vi "parse url.vi"(11 "connection string in":string) -> (1 "service":string, 2 "port":u16, 3 "net address":u32)   [LabVIEW 2015]
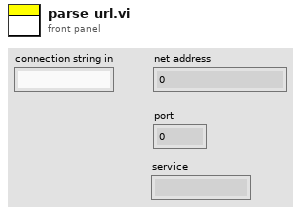
[diagram p1: front panel]
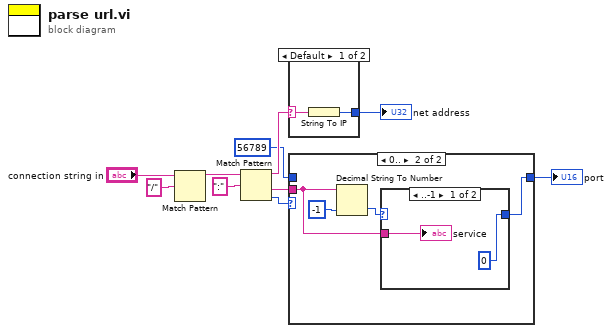
[diagram p0: block diagram]
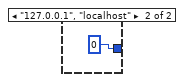
[diagram p2: hidden frame]
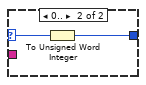
[diagram p4: hidden frame]
diagram:
  n1 = Match Pattern(string="connection string in", regular expression="/") -> (before substring=w7:string)  [unwired: 1 in, 3 out]
  n2 = Match Pattern(string=w7, regular expression=":") -> (before substring=w9:string, after substring=w3:string, offset past match=w2:i32)  [unwired: 1 in, 1 out]
  n3 = case shown="Default" w9 {
    selector: w9 -> [w12 _]
    tunnel: [w11 u32 0 ("net address")] -> w10
    frame Default {
      n4 = String To IP(1:w12) -> (0:w11:u32)
    }
    frame "127.0.0.1", "localhost" {
    }
  }
  "net address" <- w10
  n5 = case shown="0.." w2 {
    tunnel: w3 -> [_ w15]
    tunnel: [w14 w16] -> w4
    tunnel: u16 56789 ("port") -> [w14 _]
    frame ..-1 {
    }
    frame 0.. {
      n6 = Decimal String To Number(string=w15, default (0L)=-1 ("default (0 I32)")) -> (number=w17:i32)  [unwired: 1 in, 1 out]
      n7 = case shown="..-1" w17 {
        selector: w17 -> [_ w22]
        tunnel: [u16 0 w21] -> w16
        tunnel: w15 -> [w19 _]
        frame ..-1 {
          "service" <- w19
        }
        frame 0.. {
          n8 = To Unsigned Word Integer(number=w22) -> (unsigned 16bit integer=w21:u16)
        }
      }
    }
  }
  "port" <- w4
